vi "Analog_input_ch1_NSamples.vi"() -> ()   [LabVIEW 2019]
uses:
  <vilib>/Waveform/WDTFileIO.llb/Export Waveforms To Spreadsheet File (1D).vi
panel:
  out "Waveform Chart":dynamicdata(graph)
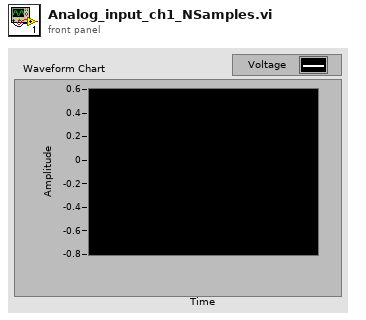
[diagram p1: front panel]
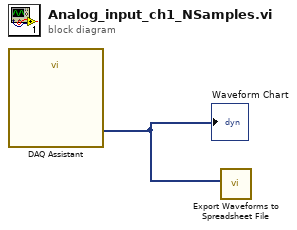
[diagram p0: block diagram]
diagram:
  n1 = call "DAQ Assistant"() -> ("data"=w1:dynamicdata)  [unwired: 17 in, 2 out]
  "Waveform Chart" <- w1
  n2 = call-poly <vilib>:"Export Waveforms to Spreadsheet File.vi"("waveforms"=w1) -> ()  [unwired: 9 in, 2 out]
